vi "TestReport_FGV.vi"(7 "ModReport":T1, 8 "Error in":errorcluster, 11 "Parameter":variant) -> (0 "Error out":errorcluster)   [LabVIEW 2016]
uses:
  TestReport_mods.ctl
  TestReport_data.ctl
  WorReport_imageData.ctl
  WorReport_tableData.ctl
  <vilib>/Utility/NIReport.llb/NI_report.lvclass
  TestReport_NumPoints.ctl
  <vilib>/Utility/NIReport.llb/HTML Report Image Alignment.ctl
  <vilib>/addons/_office/word.llb/Word Edit Cell ([str]).vi
  <vilib>/Utility/NIReport.llb/Append Image to Report (path wrap).vi
  <vilib>/addons/_office/word.llb/Word Find & Replace (str).vi
  <vilib>/addons/_office/NI_ReportGenerationToolkit.lvlib
  <vilib>/Utility/NIReport.llb/Word/NI_Word.lvclass
  <vilib>/Utility/NIReport.llb/NI_ReportGenerationCore.lvlib
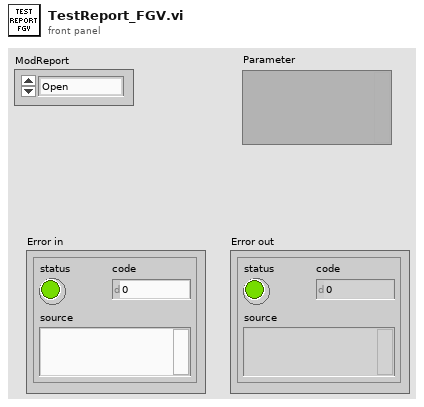
[diagram p1: front panel]
types:
  T1 = typedef "TestReport_mods.ctl" = enum16{"Open", "Table", "Image", "Tag", "ResizeAll", "Close"}
  T2 = typedef "TestReport_NumPoints.ctl" = enum16{"5 pontos", "6 pontos"}
  T3 = typedef "TestReport_data.ctl" = cluster{"ImageData":T4[], "TableData":T5[], "report":refnum<class "NI_report.lvclass">, "Resized":bool}
  T4 = typedef "WorReport_imageData.ctl" = cluster{"PathImage":path, "Legend":string}
  T5 = typedef "WorReport_tableData.ctl" = cluster{"Title":string, "ColumHeaders":string[], "Data":string[][]}
  T6 = enum16{"Standard Report", "HTML", "Word", "Excel"}
  T7 = cluster{"position (Excel)":cluster{"row":i32, "column":i32}, "name (Excel)":string, "bookmark (Word)":string}
  T8 = typedef "NI_ReportGenerationCore.lvlib/HTML Report Image Alignment.ctl" = enum16{"(default)", "LEFT", "RIGHT", "TOP", "TEXTTOP", "MIDDLE", "ABSMIDDLE", "BASELINE", "BOTTOM", "ABSBOTTOM"}
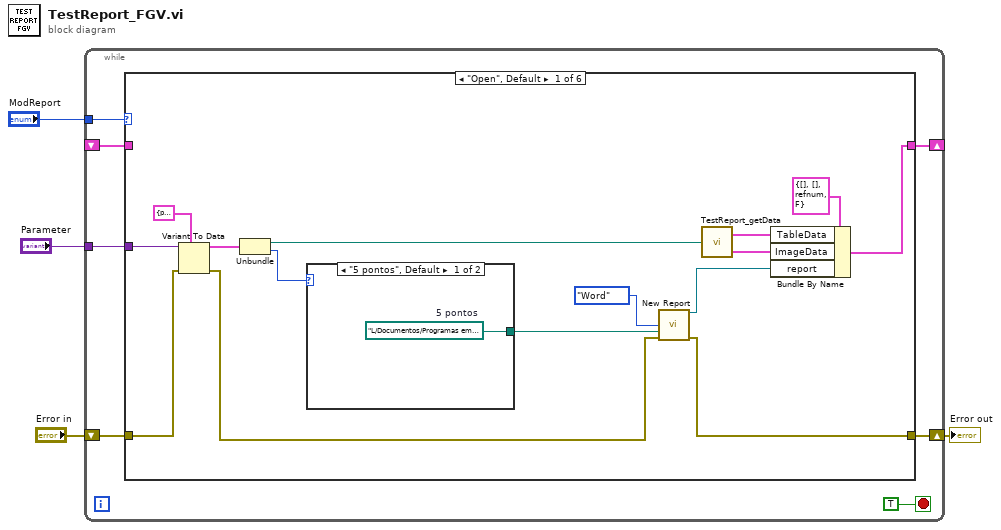
[diagram p0: block diagram]
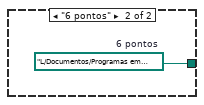
[diagram p2: hidden frame]
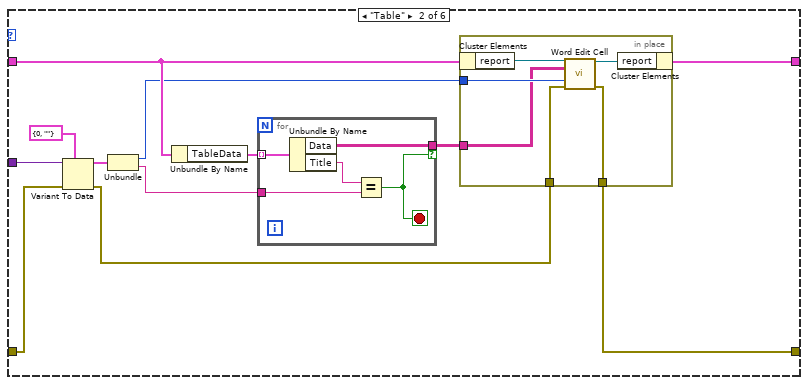
[diagram p3: hidden frame]
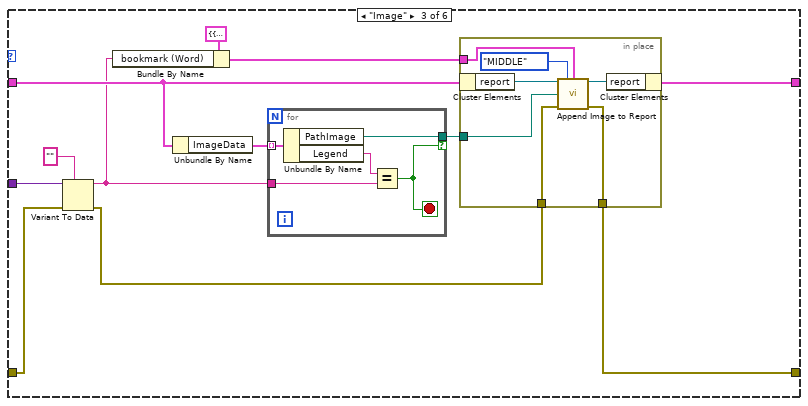
[diagram p4: hidden frame]
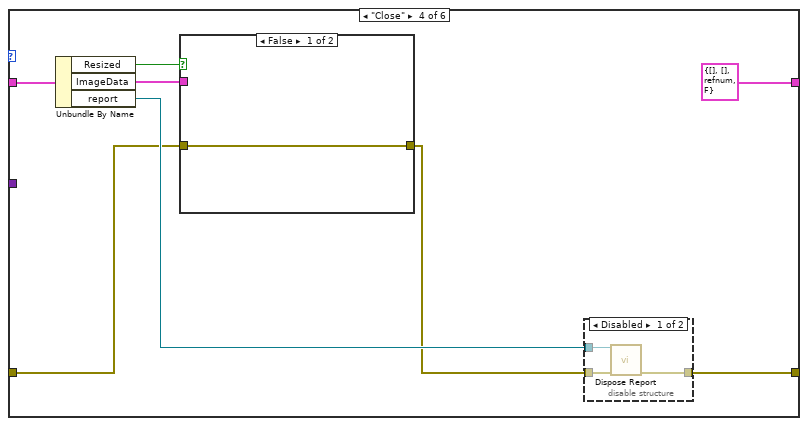
[diagram p5: hidden frame]
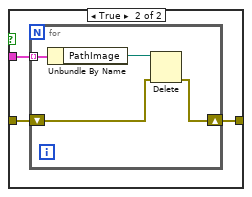
[diagram p6: hidden frame]
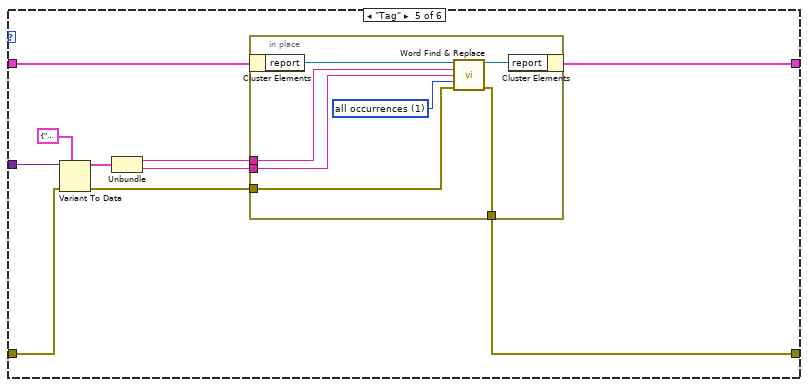
[diagram p8: hidden frame]
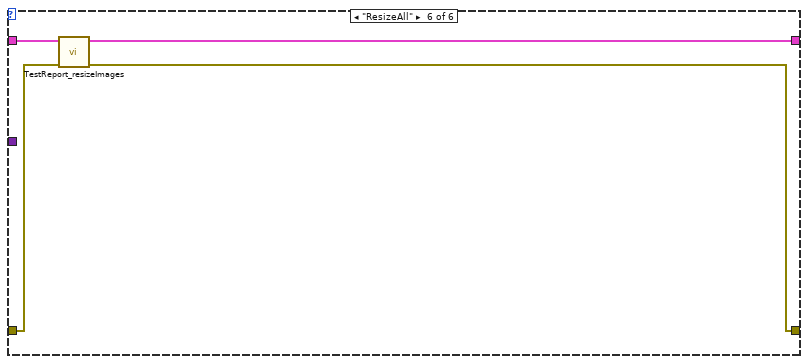
[diagram p9: hidden frame]
diagram:
  n1 = while {
    tunnel: "ModReport" -> [w10]
    shift-right: [w8] -> w2
    shift-left: "Error in" -> [w9]
    shift-right: [w7] -> _
    shift-left: _ -> [w6]
    tunnel: "Parameter" -> [w5]
    stop <- TRUE stop-if-true
    n2 = case shown="\"Open\", Default" w10 {
      tunnel: w9 -> [w25 w34 w57 w77 w102 w114]
      tunnel: [w22 w40 w63 w83 w95 w113] -> w8
      tunnel: [w19 w39 w62 T3 {"ImageData"=[], "TableData"=[], "report"=refnum, "Resized"=FALSE} ("TestReport_data") w96 w112] -> w7
      tunnel: w6 -> [_ w38 w61 w82 w104 w115]
      tunnel: w5 -> [w17 w35 w58 _ w103 _]
      frame "Open", Default {
        n3 = Variant To Data(error in=w25, type=cluster{"Report path":path, "Tipo":T2} {"Report path"=path "", "Tipo"=enum."5 pontos"} ("output cluster"), Variant=w17) -> (data=w15:cluster{"Report path":path, "Tipo":T2}, error out=w24:errorcluster)
        n4 = Unbundle(w15) -> ("Report path"=w14:path, "Tipo"=w13:T2)
        n5 = case shown="\"5 pontos\", Default" w13 {
          tunnel: [w27 w28] -> w12
          frame "5 pontos", Default {
            w27 = path "L:/Documentos/Programas em LabVIEW/Programas funcionais/PipeStressDistribution/Code/WordReport/Model - 5 pontos.docx"  # 5 pontos
          }
          frame "6 pontos" {
            w28 = path "L:/Documentos/Programas em LabVIEW/Programas funcionais/PipeStressDistribution/Code/WordReport/Model - 6 pontos.docx"  # 6 pontos
          }
        }
        n6 = call <vilib>:"New Report.vi"("report type"=T6."Word", "template (empty)"=w12, "error in (no error)"=w24) -> ("report out"=w18:refnum<class "NI_report.lvclass">, "error out"=w22:errorcluster)  [unwired: 11 in]
        n7 = call "TestReport_getData.vi"("ReportPath"=w14) -> ("TableData"=w21:T5[], "ImageData"=w20:T4[])
        n8 = Bundle By Name(cluster=T3 {"ImageData"=[], "TableData"=[], "report"=refnum, "Resized"=FALSE} ("TestReport_data"), "TableData"=w21, "ImageData"=w20, "report"=w18) -> (w19:T3)
      }
      frame "Table" {
        n9 = Variant To Data(error in=w34, type=cluster{i16, string} {0, ""}, Variant=w35) -> (data=w32:cluster{i16, string}, error out=w29:errorcluster)
        n10 = Unbundle(w32) -> (w31:i16, w30:string)
        n11 = Unbundle By Name(w38) -> ("TableData"=w37:T5[])
        n12 = for {
          tunnel: w37 -> [w45] mode=indexing
          tunnel: w30 -> [w43]
          tunnel: [w42] -> w36 if=w41
          stop <- w41 stop-if-true
          n13 = Unbundle By Name(w45) -> ("Data"=w42:string[][], "Title"=w44:string)
          n14 = Equal?(x=w44, y=w43) -> (x = y?=w41:bool)
        }
        n15 = in-place {
          in-place-border: w29 -> [w51]
          in-place-border: [w50] -> w40
          in-place-border: w31 -> [w49]
          in-place-border: w36 -> [w46]
          n16 = in-place-cluster #1(w38) -> ("report"=w48:refnum<class "NI_report.lvclass">)
          n17 = call-poly <vilib>:"Word Edit Cell.vi"("report in"=w48, "value"=w46, "table index (-1)"=w49, "error in (no error)"=w51) -> ("report out"=w47:refnum<class "NI_report.lvclass">, "error out"=w50:errorcluster)  [unwired: 10 in]
          n18 = in-place-cluster #1("report"=w47) -> (w39:T3)
        }
      }
      frame "Image" {
        n19 = Variant To Data(error in=w57, type="", Variant=w58) -> (data=w53:string, error out=w56:errorcluster)
        n20 = Bundle By Name(cluster=T7 {"position (Excel)"={"row"=0, "column"=0}, "name (Excel)"="", "bookmark (Word)"=""} ("MS Office parameters"), "bookmark (Word)"=w53) -> (w52:T7)
        n21 = Unbundle By Name(w61) -> ("ImageData"=w60:T4[])
        n22 = for {
          tunnel: w60 -> [w68] mode=indexing
          tunnel: w53 -> [w66]
          tunnel: [w65] -> w59 if=w64
          stop <- w64 stop-if-true
          n23 = Unbundle By Name(w68) -> ("PathImage"=w65:path, "Legend"=w67:string)
          n24 = Equal?(x=w67, y=w66) -> (x = y?=w64:bool)
        }
        n25 = in-place {
          in-place-border: w56 -> [w73]
          in-place-border: [w72] -> w63
          in-place-border: w59 -> [w74]
          in-place-border: w52 -> [w69]
          n26 = in-place-cluster #2(w61) -> ("report"=w75:refnum<class "NI_report.lvclass">)
          n27 = call-poly <vilib>:"Append Image to Report.vi"("report in"=w75, "alignment (default)"=HTML_Report_Image_Alignment."MIDDLE", "MS Office parameters"=w69, "path or URL of image"=w74, "error in (no error)"=w73) -> ("report out"=w71:refnum<class "NI_report.lvclass">, "error out"=w72:errorcluster)  [unwired: 7 in, 2 out]
          n28 = in-place-cluster #2("report"=w71) -> (w62:T3)
        }
      }
      frame "Close" {
        n29 = Unbundle By Name(w82) -> ("Resized"=w79:bool, "ImageData"=w78:T4[], "report"=w81:refnum<class "NI_report.lvclass">)
        n30 = case shown="False" w79 {
          tunnel: w78 -> [_ w87]
          tunnel: w77 -> [w84 w86]
          tunnel: [w84 w85] -> w76
          frame False {
          }
          frame True {
            n31 = for {
              tunnel: w87 -> [w91] mode=indexing
              shift-right: [w88] -> w85
              shift-left: w86 -> [w89]
              n32 = Unbundle By Name(w91) -> ("PathImage"=w90:path)
              n33 = Delete(path (use dialog)=w90, error in=w89) -> (error out=w88:errorcluster)  [unwired: 3 in, 2 out]
            }
          }
        }
        n34 = disable-structure shown="Disabled" {
          disable-tunnel: w76 -> [w94 _]
          disable-tunnel: [w93 _] -> w83
          disable-tunnel: w81 -> [w92 _]
          frame Disabled {
            n35 = call-dynamic "Dispose Report.vi"("report in"=w92, "error in (no error)"=w94) -> ("error out"=w93:errorcluster)  [unwired: 13 in]
          }
          frame Enabled {
          }
        }
      }
      frame "Tag" {
        n36 = Variant To Data(error in=w102, type=cluster{string, string} {"", ""}, Variant=w103) -> (data=w99:cluster{string, string}, error out=w101:errorcluster)
        n37 = Unbundle(w99) -> (w98:string, w97:string)
        n38 = in-place {
          in-place-border: w101 -> [w109]
          in-place-border: w98 -> [w108]
          in-place-border: w97 -> [w107]
          in-place-border: [w105] -> w95
          w106 = u16 1 items=["first occurrence", "all occurrences"] ("search scope (first occurrence)")
          n39 = in-place-cluster #3(w104) -> ("report"=w111:refnum<class "NI_report.lvclass">)
          n40 = call-poly <vilib>:"Word Find & Replace.vi"("report in"=w111, "find what?"=w108, "replace with"=w107, "search scope (first occurrence)"=w106, "error in (no error)"=w109) -> ("report out"=w110:refnum<class "NI_report.lvclass">, "error out"=w105:errorcluster)  [unwired: 8 in, 1 out]
          n41 = in-place-cluster #3("report"=w110) -> (w96:T3)
        }
      }
      frame "ResizeAll" {
        n42 = call "TestReport_resizeImages.vi"("error in (no error)"=w114, "TestReport_data in"=w115) -> ("error out"=w113:errorcluster, "TestReport_data out"=w112:T3)  [unwired: 8 in]
      }
    }
  }
  "Error out" <- w2
